vi "2 angle_difference_sign.vi"(1 "Angle 2":dbl, 2 "Angle 1":dbl) -> (0 "Difference":dbl)   [LabVIEW 2011]
doc: "Returns the angle between to headings, accounting for wraparound (0 and 355 are 5 degrees apart)"
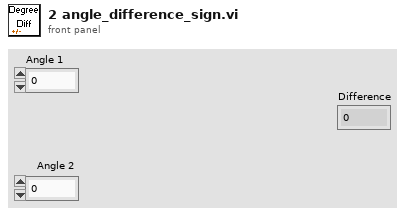
[diagram p1: front panel]
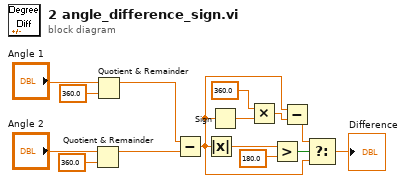
[diagram p0: block diagram]
diagram:
  n1 = Quotient & Remainder(x="Angle 2", y=360.0) -> (x-y*floor(x/y)=w1:dbl)  [unwired: 1 out]
  n2 = Quotient & Remainder(x="Angle 1", y=360.0) -> (x-y*floor(x/y)=w5:dbl)  [unwired: 1 out]
  n3 = Subtract(x=w5, y=w1) -> (x-y=w8:dbl)
  n4 = Absolute Value(x=w8) -> (abs(x)=w14:dbl)
  n5 = Sign(1:w8) -> (0:w11:dbl)
  n6 = Multiply(x=360.0 ("y"), y=w11) -> (x*y=w7:dbl)
  n7 = Greater?(x=w14, y=180.0) -> (0:w15:bool)
  n8 = Subtract(x=w8, y=w7) -> (x-y=w9:dbl)
  n9 = Select(t=w9, s=w15, f=w8) -> (s? t:f=→"Difference":dbl)
